vi "Lab Panel V5.22.1.vi"() -> ()   [LabVIEW 2013] (continued)
                                n836 = Number To Decimal String(number=w1475) -> (decimal integer string=w1488:string)  [unwired: 1 in]
                                n837 = Build Array(w1479, w1478, w1490, w1489, w1488) -> (w1487:string[])
                                n838 = TDMS Set Properties(5:w1487, 7:w1481, 11:w1491) -> ()  [unwired: 3 in, 4 out]
                              }
                              frame #3 {
                                n839 = local read "DISP LAB03-2"() -> (w1496:T4)
                                n840 = Concatenate Strings("LAB03-2  ", w1495) -> (w1497:string)
                                n841 = Two Button Dialog(message=w1497, 1:w1493, 2:w1494) -> (T button?=w1499:bool)
                                n842 = case shown="True" w1499 {
                                tunnel: w1496 -> [w1506 w1507]
                                tunnel: [w1506 w1507] -> w1503
                                tunnel: [w1505 w1508] -> w1502
                                tunnel: [w1504 w1508] -> w1501
                                frame False {
                                n843 = Unbundle(w1506) -> ("CYCLE"=w1505:dbl, "MINS"=w1504:dbl)  [unwired: 1 out]
                                }
                                frame True {
                                w1508 = 0.0
                                }
                                }
                                n844 = Bundle(cluster=w1503, "CYCLE"=w1502, "MINS"=w1501, "STATUS"="RUN") -> (w1492:T4)
                                n845 = local write "DISP LAB03-2"(w1492) -> ()
                              }
                              frame #4 {
                                n846 = local read "TEMP START LAB03-2"() -> (w1511:cluster{"TL":dbl, "TN":dbl})
                                n847 = Bundle(cluster=w1511, "TL"=w1509, "TN"=w1509) -> (w1510:cluster{"TL":dbl, "TN":dbl})
                                n848 = local write "TEMP START LAB03-2"(w1510) -> ()
                              }
                            }
                          }
                        }
                      }
                    }
                  }
                }
              }
              event "RUN LAB04-1": Value Change {
                n849 = event-data() -> ("NewVal"=w1516:bool)  [unwired: 1 in, 5 out]
                n850 = local write "run lab04-1"(w1516) -> ()
                n851 = case shown="True" w1516 {
                  tunnel: w1522 -> [_ w1560]
                  tunnel: w1521 -> [_ w1559]
                  tunnel: w1519 -> [w1524 w1558]
                  tunnel: w1520 -> [_ w1557]
                  tunnel: w1518 -> [_ w1556]
                  tunnel: [w1523 w1555] -> w1517
                  tunnel: w1515 -> [_ w1554]
                  tunnel: w1514 -> [_ w1553]
                  tunnel: w1513 -> [_ w1552]
                  tunnel: w1512 -> [_ w1550]
                  frame False {
                    # "stop test"
                    n852 = stacked-sequence {
                      tunnel: w1524 -> [w1533 _]
                      tunnel: [w1525 _] -> w1523
                      frame #0 {
                        n853 = local read "DISP LAB04-1"() -> (w1532:T4)
                        n854 = Unbundle(w1532) -> ("CYCLE"=w1530:dbl, "MINS"=w1531:dbl)  [unwired: 1 out]
                        n855 = case shown="\"CYCLE TEST\"" w1533 {
                          tunnel: w1531 -> [_ _ w1540]
                          tunnel: w1530 -> [w1538 w1539 _]
                          tunnel: [w1538 w1539 w1540] -> w1529
                          frame "CHART TEST", Default {
                          }
                          frame "CYCLE TEST" {
                          }
                          frame "T-RISE TEST" {
                          }
                        }
                        n856 = local read "TDMS LAB04-1"() -> (w1537:refnum<k34>)
                        n857 = Build Array("STOPPED") -> (w1534:string[])
                        n858 = Build Array(w1529) -> (w1528:dbl[])
                        n859 = TDMS Write(0:w1537, 5:"TEST RESULT", 7:w1534, 9:w1528) -> (4:w1526:refnum<k34>, 15:w1527:errorcluster)  [unwired: 2 in, 2 out]
                        n860 = TDMS Close(8:w1527, 11:w1526) -> (0:w1525:errorcluster)  [unwired: 1 out]
                      }
                      frame #1 {
                        n861 = local read "DISP LAB04-1"() -> (w1544:T4)
                        n862 = stacked-sequence {
                          tunnel: "LAB04-1" -> [w1546 w1548]
                          frame #0 {
                            n863 = call "sub vi - defrag tdms v1.vi"("panel id"=w1546) -> ("error out"=w1545:errorcluster)  [unwired: 10 in]
                            n864 = local write "data file error"(w1545) -> ()
                          }
                          frame #1 {
                            n865 = call "Save data file (stop) v3.vi"("panel id"=w1548) -> ("network file save error"=w1547:errorcluster)  [unwired: 9 in, 1 out]
                            n866 = local write "RESULT LAB04-1"(FALSE) -> ()
                            n867 = local write "data file error"(w1547) -> ()
                          }
                        }
                        n868 = Bundle(cluster=w1544, "STATUS"="STOP") -> (w1542:T4)  [unwired: 2 in]
                        n869 = local write "DISP LAB04-1"(w1542) -> ()
                      }
                    }
                  }
                  frame True {
                    n870 = local read "SIG LAB04-1"() -> (w1551:T2)
                    n871 = stacked-sequence {
                      seq-local: [w1562 _] -> [_ w1566]
                      tunnel: w1560 -> [_ w1576]
                      tunnel: w1559 -> [_ w1575]
                      tunnel: w1558 -> [_ w1574]
                      tunnel: w1557 -> [_ w1573]
                      tunnel: w1556 -> [_ w1572]
                      tunnel: [_ w1571] -> w1555
                      tunnel: w1554 -> [_ w1570]
                      tunnel: w1553 -> [_ w1569]
                      tunnel: w1552 -> [_ w1568]
                      tunnel: w1551 -> [w1561 w1567]
                      tunnel: w1550 -> [_ w1565]
                      frame #0 {
                        n872 = Unbundle(w1561) -> ("AMPS"=w1564:dbl)  [unwired: 4 out]
                        n873 = call "Check For Amps on v1.vi"("ID"="LAB04-1", "amps"=w1564) -> ("amps"=w1562:bool)  [unwired: 9 in]
                      }
                      frame #1 {
                        n874 = case shown="True" w1566 {
                          tunnel: w1576 -> [_ w1589]
                          tunnel: w1575 -> [_ w1588]
                          tunnel: w1574 -> [_ w1587]
                          tunnel: w1573 -> [_ w1586]
                          tunnel: w1572 -> [_ w1585]
                          tunnel: [errorcluster {"status"=FALSE, "code"=0, "source"=""} ("error out") w1584] -> w1571
                          tunnel: w1570 -> [_ w1583]
                          tunnel: w1569 -> [_ w1582]
                          tunnel: w1568 -> [_ w1581]
                          tunnel: w1567 -> [_ w1580]
                          tunnel: w1565 -> [_ w1579]
                          frame False {
                            w1577 = FALSE
                            n875 = local write "RUN LAB04-1"(w1577) -> ()
                            n876 = local write "run lab04-1"(w1577) -> ()
                          }
                          frame True {
                            n877 = stacked-sequence {
                              seq-local: [w1590 _ _ _ _] -> [_ w1614 _ _ _]
                              tunnel: w1589 -> [w1595 _ _ _ _]
                              tunnel: w1588 -> [w1591 _ _ _ _]
                              tunnel: w1587 -> [w1605 _ _ _ _]
                              tunnel: w1586 -> [w1598 _ _ _ _]
                              tunnel: w1585 -> [w1593 _ _ _ _]
                              tunnel: [_ w1609 _ _ _] -> w1584
                              tunnel: w1583 -> [_ _ _ w1635 _]
                              tunnel: w1582 -> [_ _ _ w1634 _]
                              tunnel: w1581 -> [_ _ _ w1633 _]
                              tunnel: w1580 -> [_ _ _ _ _]
                              tunnel: w1579 -> [_ _ _ _ w1649]
                              frame #0 {
                                w1592 = "\\"
                                n878 = local read "SET LAB04-1"() -> (w1600:T5)
                                n879 = case shown="\"CYCLE TEST\"" w1605 {
                                tunnel: ["L04-1-CHART TEST-" "L04-1-CYCLE TEST-" "L04-1-T-RISE TEST-"] -> w1601
                                frame "CHART TEST", Default {
                                }
                                frame "CYCLE TEST" {
                                }
                                frame "T-RISE TEST" {
                                }
                                }
                                n880 = Unbundle(w1600) -> ("DESCRIPTION"=w1599:string)  [unwired: 4 out]
                                n881 = Concatenate Strings(w1595, "\\", w1593, w1592, w1591, w1592) -> (w1602:string)
                                n882 = String To Path(string=w1602) -> (path=w1604:path)
                                n883 = Concatenate Strings(w1602, w1601, w1599, "-", w1598, ".tdms") -> (w1590:string)
                                n884 = Create Folder(path (use dialog)=w1604) -> (error out=w1603:errorcluster)  [unwired: 2 in, 2 out]
                                n885 = global write "Global 1.vi" "LAB04-1 FILE"(w1590) -> ()
                                n886 = call <vilib>:"Clear Errors.vi"("error in (no error)"=w1603) -> ()  [unwired: 6 in, 1 out]
                              }
                              frame #1 {
                                (unwired) FALSE
                                n887 = String To Path(string=w1614) -> (path=w1610:path)
                                n888 = TDMS Open(6:FALSE, 10:T21."create or replace" ("operation (0:open)"), 11:w1610) -> (0:w1609:errorcluster, 3:→"TDMS LAB04-1":refnum<k34>)  [unwired: 4 in]
                              }
                              frame #2 {
                                n889 = local read "SET LAB04-1"() -> (w1620:T5)
                                n890 = local read "TDMS LAB04-1"() -> (w1631:refnum<k34>)
                                n891 = Build Array("Testers Name", "Description", "Set Test Cycles", "T-Rise minutes", "T-Rise Deg C") -> (w1621:string[])
                                n892 = Unbundle(w1620) -> ("NAME"=w1619:string, "DESCRIPTION"=w1618:string, "CYCLES"=w1617:dbl, "T-RISE mins"=w1616:dbl, "T-RISE deg C"=w1615:dbl)
                                n893 = Number To Decimal String(number=w1617) -> (decimal integer string=w1630:string)  [unwired: 1 in]
                                n894 = Number To Decimal String(number=w1616) -> (decimal integer string=w1629:string)  [unwired: 1 in]
                                n895 = Number To Decimal String(number=w1615) -> (decimal integer string=w1628:string)  [unwired: 1 in]
                                n896 = Build Array(w1619, w1618, w1630, w1629, w1628) -> (w1627:string[])
                                n897 = TDMS Set Properties(5:w1627, 7:w1621, 11:w1631) -> ()  [unwired: 3 in, 4 out]
                              }
                              frame #3 {
                                n898 = local read "DISP LAB04-1"() -> (w1636:T4)
                                n899 = Concatenate Strings("LAB04-1  ", w1635) -> (w1637:string)
                                n900 = Two Button Dialog(message=w1637, 1:w1633, 2:w1634) -> (T button?=w1639:bool)
                                n901 = case shown="True" w1639 {
                                tunnel: w1636 -> [w1646 w1647]
                                tunnel: [w1646 w1647] -> w1643
                                tunnel: [w1645 w1648] -> w1642
                                tunnel: [w1644 w1648] -> w1641
                                frame False {
                                n902 = Unbundle(w1646) -> ("CYCLE"=w1645:dbl, "MINS"=w1644:dbl)  [unwired: 1 out]
                                }
                                frame True {
                                w1648 = 0.0
                                }
                                }
                                n903 = Bundle(cluster=w1643, "CYCLE"=w1642, "MINS"=w1641, "STATUS"="RUN") -> (w1632:T4)
                                n904 = local write "DISP LAB04-1"(w1632) -> ()
                              }
                              frame #4 {
                                n905 = local read "TEMP START LAB04-1"() -> (w1651:cluster{"TL":dbl, "TN":dbl})
                                n906 = Bundle(cluster=w1651, "TL"=w1649, "TN"=w1649) -> (w1650:cluster{"TL":dbl, "TN":dbl})
                                n907 = local write "TEMP START LAB04-1"(w1650) -> ()
                              }
                            }
                          }
                        }
                      }
                    }
                  }
                }
              }
              event "RUN LAB04-2": Value Change {
                n908 = event-data() -> ("NewVal"=w1656:bool)  [unwired: 1 in, 5 out]
                n909 = local write "run lab04-2"(w1656) -> ()
                n910 = case shown="True" w1656 {
                  tunnel: w1662 -> [_ w1700]
                  tunnel: w1661 -> [_ w1699]
                  tunnel: w1659 -> [w1664 w1698]
                  tunnel: w1660 -> [_ w1697]
                  tunnel: w1658 -> [_ w1696]
                  tunnel: [w1663 w1695] -> w1657
                  tunnel: w1655 -> [_ w1694]
                  tunnel: w1654 -> [_ w1693]
                  tunnel: w1653 -> [_ w1692]
                  tunnel: w1652 -> [_ w1690]
                  frame False {
                    # "stop test"
                    n911 = stacked-sequence {
                      tunnel: w1664 -> [w1673 _]
                      tunnel: [w1665 _] -> w1663
                      frame #0 {
                        n912 = local read "DISP LAB04-2"() -> (w1672:T4)
                        n913 = Unbundle(w1672) -> ("CYCLE"=w1670:dbl, "MINS"=w1671:dbl)  [unwired: 1 out]
                        n914 = case shown="\"CYCLE TEST\"" w1673 {
                          tunnel: w1671 -> [_ _ w1680]
                          tunnel: w1670 -> [w1678 w1679 _]
                          tunnel: [w1678 w1679 w1680] -> w1669
                          frame "CHART TEST", Default {
                          }
                          frame "CYCLE TEST" {
                          }
                          frame "T-RISE TEST" {
                          }
                        }
                        n915 = local read "TDMS LAB04-2"() -> (w1677:refnum<k34>)
                        n916 = Build Array("STOPPED") -> (w1674:string[])
                        n917 = Build Array(w1669) -> (w1668:dbl[])
                        n918 = TDMS Write(0:w1677, 5:"TEST RESULT", 7:w1674, 9:w1668) -> (4:w1666:refnum<k34>, 15:w1667:errorcluster)  [unwired: 2 in, 2 out]
                        n919 = TDMS Close(8:w1667, 11:w1666) -> (0:w1665:errorcluster)  [unwired: 1 out]
                      }
                      frame #1 {
                        n920 = local read "DISP LAB04-2"() -> (w1684:T4)
                        n921 = stacked-sequence {
                          tunnel: "LAB04-2" -> [w1686 w1688]
                          frame #0 {
                            n922 = call "sub vi - defrag tdms v1.vi"("panel id"=w1686) -> ("error out"=w1685:errorcluster)  [unwired: 10 in]
                            n923 = local write "data file error"(w1685) -> ()
                          }
                          frame #1 {
                            n924 = call "Save data file (stop) v3.vi"("panel id"=w1688) -> ("network file save error"=w1687:errorcluster)  [unwired: 9 in, 1 out]
                            n925 = local write "RESULT LAB04-2"(FALSE) -> ()
                            n926 = local write "data file error"(w1687) -> ()
                          }
                        }
                        n927 = Bundle(cluster=w1684, "STATUS"="STOP") -> (w1682:T4)  [unwired: 2 in]
                        n928 = local write "DISP LAB04-2"(w1682) -> ()
                      }
                    }
                  }
                  frame True {
                    n929 = local read "SIG LAB04-2"() -> (w1691:T2)
                    n930 = stacked-sequence {
                      seq-local: [w1702 _] -> [_ w1706]
                      tunnel: w1700 -> [_ w1716]
                      tunnel: w1699 -> [_ w1715]
                      tunnel: w1698 -> [_ w1714]
                      tunnel: w1697 -> [_ w1713]
                      tunnel: w1696 -> [_ w1712]
                      tunnel: [_ w1711] -> w1695
                      tunnel: w1694 -> [_ w1710]
                      tunnel: w1693 -> [_ w1709]
                      tunnel: w1692 -> [_ w1708]
                      tunnel: w1691 -> [w1701 w1707]
                      tunnel: w1690 -> [_ w1705]
                      frame #0 {
                        n931 = Unbundle(w1701) -> ("AMPS"=w1704:dbl)  [unwired: 4 out]
                        n932 = call "Check For Amps on v1.vi"("ID"="LAB04-2", "amps"=w1704) -> ("amps"=w1702:bool)  [unwired: 9 in]
                      }
                      frame #1 {
                        n933 = case shown="True" w1706 {
                          tunnel: w1716 -> [_ w1729]
                          tunnel: w1715 -> [_ w1728]
                          tunnel: w1714 -> [_ w1727]
                          tunnel: w1713 -> [_ w1726]
                          tunnel: w1712 -> [_ w1725]
                          tunnel: [errorcluster {"status"=FALSE, "code"=0, "source"=""} ("error out") w1724] -> w1711
                          tunnel: w1710 -> [_ w1723]
                          tunnel: w1709 -> [_ w1722]
                          tunnel: w1708 -> [_ w1721]
                          tunnel: w1707 -> [_ w1720]
                          tunnel: w1705 -> [_ w1719]
                          frame False {
                            w1717 = FALSE
                            n934 = local write "RUN LAB04-2"(w1717) -> ()
                            n935 = local write "run lab04-2"(w1717) -> ()
                          }
                          frame True {
                            n936 = stacked-sequence {
                              seq-local: [w1730 _ _ _ _] -> [_ w1754 _ _ _]
                              tunnel: w1729 -> [w1735 _ _ _ _]
                              tunnel: w1728 -> [w1731 _ _ _ _]
                              tunnel: w1727 -> [w1745 _ _ _ _]
                              tunnel: w1726 -> [w1738 _ _ _ _]
                              tunnel: w1725 -> [w1733 _ _ _ _]
                              tunnel: [_ w1749 _ _ _] -> w1724
                              tunnel: w1723 -> [_ _ _ w1775 _]
                              tunnel: w1722 -> [_ _ _ w1774 _]
                              tunnel: w1721 -> [_ _ _ w1773 _]
                              tunnel: w1720 -> [_ _ _ _ _]
                              tunnel: w1719 -> [_ _ _ _ w1789]
                              frame #0 {
                                w1732 = "\\"
                                n937 = local read "SET LAB04-2"() -> (w1740:T5)
                                n938 = case shown="\"CHART TEST\", Default" w1745 {
                                tunnel: ["L04-2-CHART TEST-" "L04-2-CYCLE TEST-" "L04-2-T-RISE TEST-"] -> w1741
                                frame "CHART TEST", Default {
                                }
                                frame "CYCLE TEST" {
                                }
                                frame "T-RISE TEST" {
                                }
                                }
                                n939 = Unbundle(w1740) -> ("DESCRIPTION"=w1739:string)  [unwired: 4 out]
                                n940 = Concatenate Strings(w1735, "\\", w1733, w1732, w1731, w1732) -> (w1742:string)
                                n941 = String To Path(string=w1742) -> (path=w1744:path)
                                n942 = Concatenate Strings(w1742, w1741, w1739, "-", w1738, ".tdms") -> (w1730:string)
                                n943 = Create Folder(path (use dialog)=w1744) -> (error out=w1743:errorcluster)  [unwired: 2 in, 2 out]
                                n944 = global write "Global 1.vi" "LAB04-2 FILE"(w1730) -> ()
                                n945 = call <vilib>:"Clear Errors.vi"("error in (no error)"=w1743) -> ()  [unwired: 6 in, 1 out]
                              }
                              frame #1 {
                                (unwired) FALSE
                                n946 = String To Path(string=w1754) -> (path=w1750:path)
                                n947 = TDMS Open(6:FALSE, 10:T21."create or replace" ("operation (0:open)"), 11:w1750) -> (0:w1749:errorcluster, 3:→"TDMS LAB04-2":refnum<k34>)  [unwired: 4 in]
                              }
                              frame #2 {
                                n948 = local read "SET LAB04-2"() -> (w1760:T5)
                                n949 = local read "TDMS LAB04-2"() -> (w1771:refnum<k34>)
                                n950 = Build Array("Testers Name", "Description", "Set Test Cycles", "T-Rise minutes", "T-Rise Deg C") -> (w1761:string[])
                                n951 = Unbundle(w1760) -> ("NAME"=w1759:string, "DESCRIPTION"=w1758:string, "CYCLES"=w1757:dbl, "T-RISE mins"=w1756:dbl, "T-RISE deg C"=w1755:dbl)
                                n952 = Number To Decimal String(number=w1757) -> (decimal integer string=w1770:string)  [unwired: 1 in]
                                n953 = Number To Decimal String(number=w1756) -> (decimal integer string=w1769:string)  [unwired: 1 in]
                                n954 = Number To Decimal String(number=w1755) -> (decimal integer string=w1768:string)  [unwired: 1 in]
                                n955 = Build Array(w1759, w1758, w1770, w1769, w1768) -> (w1767:string[])
                                n956 = TDMS Set Properties(5:w1767, 7:w1761, 11:w1771) -> ()  [unwired: 3 in, 4 out]
                              }
                              frame #3 {
                                n957 = local read "DISP LAB04-2"() -> (w1776:T4)
                                n958 = Concatenate Strings("LAB04-2 ", w1775) -> (w1777:string)
                                n959 = Two Button Dialog(message=w1777, 1:w1773, 2:w1774) -> (T button?=w1779:bool)
                                n960 = case shown="True" w1779 {
                                tunnel: w1776 -> [w1786 w1787]
                                tunnel: [w1786 w1787] -> w1783
                                tunnel: [w1785 w1788] -> w1782
                                tunnel: [w1784 w1788] -> w1781
                                frame False {
                                n961 = Unbundle(w1786) -> ("CYCLE"=w1785:dbl, "MINS"=w1784:dbl)  [unwired: 1 out]
                                }
                                frame True {
                                w1788 = 0.0
                                }
                                }
                                n962 = Bundle(cluster=w1783, "CYCLE"=w1782, "MINS"=w1781, "STATUS"="RUN") -> (w1772:T4)
                                n963 = local write "DISP LAB04-2"(w1772) -> ()
                              }
                              frame #4 {
                                n964 = local read "TEMP START LAB04-2"() -> (w1791:cluster{"TL":dbl, "TN":dbl})
                                n965 = Bundle(cluster=w1791, "TL"=w1789, "TN"=w1789) -> (w1790:cluster{"TL":dbl, "TN":dbl})
                                n966 = local write "TEMP START LAB04-2"(w1790) -> ()
                              }
                            }
                          }
                        }
                      }
                    }
                  }
                }
              }
              event "RUN LAB05-1": Value Change {
                n967 = event-data() -> ("NewVal"=w1796:bool)  [unwired: 1 in, 5 out]
                n968 = local write "run lab05-1"(w1796) -> ()
                n969 = case shown="True" w1796 {
                  tunnel: w1802 -> [_ w1840]
                  tunnel: w1801 -> [_ w1839]
                  tunnel: w1799 -> [w1804 w1838]
                  tunnel: w1800 -> [_ w1837]
                  tunnel: w1798 -> [_ w1836]
                  tunnel: [w1803 w1835] -> w1797
                  tunnel: w1795 -> [_ w1834]
                  tunnel: w1794 -> [_ w1833]
                  tunnel: w1793 -> [_ w1832]
                  tunnel: w1792 -> [_ w1830]
                  frame False {
                    # "stop test"
                    n970 = stacked-sequence {
                      tunnel: w1804 -> [w1813 _]
                      tunnel: [w1805 _] -> w1803
                      frame #0 {
                        n971 = local read "DISP LAB05-1"() -> (w1812:T4)
                        n972 = Unbundle(w1812) -> ("CYCLE"=w1810:dbl, "MINS"=w1811:dbl)  [unwired: 1 out]
                        n973 = case shown="\"CYCLE TEST\"" w1813 {
                          tunnel: w1811 -> [_ _ w1820]
                          tunnel: w1810 -> [w1818 w1819 _]
                          tunnel: [w1818 w1819 w1820] -> w1809
                          frame "CHART TEST", Default {
                          }
                          frame "CYCLE TEST" {
                          }
                          frame "T-RISE TEST" {
                          }
                        }
                        n974 = local read "TDMS LAB05-1"() -> (w1817:refnum<k34>)
                        n975 = Build Array("STOPPED") -> (w1814:string[])
                        n976 = Build Array(w1809) -> (w1808:dbl[])
                        n977 = TDMS Write(0:w1817, 5:"TEST RESULT", 7:w1814, 9:w1808) -> (4:w1806:refnum<k34>, 15:w1807:errorcluster)  [unwired: 2 in, 2 out]
                        n978 = TDMS Close(8:w1807, 11:w1806) -> (0:w1805:errorcluster)  [unwired: 1 out]
                      }
                      frame #1 {
                        n979 = local read "DISP LAB05-1"() -> (w1824:T4)
                        n980 = stacked-sequence {
                          tunnel: "LAB05-1" -> [w1826 w1828]
                          frame #0 {
                            n981 = call "sub vi - defrag tdms v1.vi"("panel id"=w1826) -> ("error out"=w1825:errorcluster)  [unwired: 10 in]
                            n982 = local write "data file error"(w1825) -> ()
                          }
                          frame #1 {
                            n983 = call "Save data file (stop) v3.vi"("panel id"=w1828) -> ("network file save error"=w1827:errorcluster)  [unwired: 9 in, 1 out]
                            n984 = local write "RESULT LAB05-1"(FALSE) -> ()
                            n985 = local write "data file error"(w1827) -> ()
                          }
                        }
                        n986 = Bundle(cluster=w1824, "STATUS"="STOP") -> (w1822:T4)  [unwired: 2 in]
                        n987 = local write "DISP LAB05-1"(w1822) -> ()
                      }
                    }
                  }
                  frame True {
                    n988 = local read "SIG LAB05-1"() -> (w1831:T2)
                    n989 = stacked-sequence {
                      seq-local: [w1842 _] -> [_ w1846]
                      tunnel: w1840 -> [_ w1856]
                      tunnel: w1839 -> [_ w1855]
                      tunnel: w1838 -> [_ w1854]
                      tunnel: w1837 -> [_ w1853]
                      tunnel: w1836 -> [_ w1852]
                      tunnel: [_ w1851] -> w1835
                      tunnel: w1834 -> [_ w1850]
                      tunnel: w1833 -> [_ w1849]
                      tunnel: w1832 -> [_ w1848]
                      tunnel: w1831 -> [w1841 w1847]
                      tunnel: w1830 -> [_ w1845]
                      frame #0 {
                        n990 = Unbundle(w1841) -> ("AMPS"=w1844:dbl)  [unwired: 4 out]
                        n991 = call "Check For Amps on v1.vi"("ID"="LAB05-1", "amps"=w1844) -> ("amps"=w1842:bool)  [unwired: 9 in]
                      }
                      frame #1 {
                        n992 = case shown="True" w1846 {
                          tunnel: w1856 -> [_ w1869]
                          tunnel: w1855 -> [_ w1868]
                          tunnel: w1854 -> [_ w1867]
                          tunnel: w1853 -> [_ w1866]
                          tunnel: w1852 -> [_ w1865]
                          tunnel: [errorcluster {"status"=FALSE, "code"=0, "source"=""} ("error out") w1864] -> w1851
                          tunnel: w1850 -> [_ w1863]
                          tunnel: w1849 -> [_ w1862]
                          tunnel: w1848 -> [_ w1861]
                          tunnel: w1847 -> [_ w1860]
                          tunnel: w1845 -> [_ w1859]
                          frame False {
                            w1857 = FALSE
                            n993 = local write "RUN LAB05-1"(w1857) -> ()
                            n994 = local write "run lab05-1"(w1857) -> ()
                          }
                          frame True {
                            n995 = stacked-sequence {
                              seq-local: [w1870 _ _ _ _] -> [_ w1894 _ _ _]
                              tunnel: w1869 -> [w1875 _ _ _ _]
                              tunnel: w1868 -> [w1871 _ _ _ _]
                              tunnel: w1867 -> [w1885 _ _ _ _]
                              tunnel: w1866 -> [w1878 _ _ _ _]
                              tunnel: w1865 -> [w1873 _ _ _ _]
                              tunnel: [_ w1889 _ _ _] -> w1864
                              tunnel: w1863 -> [_ _ _ w1914 _]
                              tunnel: w1862 -> [_ _ _ w1913 _]
                              tunnel: w1861 -> [_ _ _ w1912 _]
                              tunnel: w1860 -> [_ _ _ _ _]
                              tunnel: w1859 -> [_ _ _ _ w1929]
                              frame #0 {
                                w1872 = "\\"
                                n996 = local read "SET LAB05-1"() -> (w1880:T5)
                                n997 = case shown="\"CYCLE TEST\"" w1885 {
                                tunnel: ["L05-1-CHART TEST-" "L05-1-CYCLE TEST-" "L05-1-T-RISE TEST-"] -> w1881
                                frame "CHART TEST", Default {
                                }
                                frame "CYCLE TEST" {
                                }
                                frame "T-RISE TEST" {
                                }
                                }
                                n998 = Unbundle(w1880) -> ("DESCRIPTION"=w1879:string)  [unwired: 4 out]
                                n999 = Concatenate Strings(w1875, "\\", w1873, w1872, w1871, w1872) -> (w1882:string)
                                n1000 = String To Path(string=w1882) -> (path=w1884:path)
                                n1001 = Concatenate Strings(w1882, w1881, w1879, "-", w1878, ".tdms") -> (w1870:string)
                                n1002 = Create Folder(path (use dialog)=w1884) -> (error out=w1883:errorcluster)  [unwired: 2 in, 2 out]
                                n1003 = global write "Global 1.vi" "LAB05-1 FILE"(w1870) -> ()
                                n1004 = call <vilib>:"Clear Errors.vi"("error in (no error)"=w1883) -> ()  [unwired: 6 in, 1 out]
                              }
                              frame #1 {
                                (unwired) FALSE
                                n1005 = String To Path(string=w1894) -> (path=w1890:path)
                                n1006 = TDMS Open(6:FALSE, 10:T21."create or replace" ("operation (0:open)"), 11:w1890) -> (0:w1889:errorcluster, 3:→"TDMS LAB05-1":refnum<k34>)  [unwired: 4 in]
                              }
                              frame #2 {
                                n1007 = local read "SET LAB05-1"() -> (w1900:T5)
                                n1008 = local read "TDMS LAB05-1"() -> (w1911:refnum<k34>)
                                n1009 = Build Array("Testers Name", "Description", "Set Test Cycles", "T-Rise minutes", "T-Rise Deg C") -> (w1901:string[])
                                n1010 = Unbundle(w1900) -> ("NAME"=w1899:string, "DESCRIPTION"=w1898:string, "CYCLES"=w1897:dbl, "T-RISE mins"=w1896:dbl, "T-RISE deg C"=w1895:dbl)
                                n1011 = Number To Decimal String(number=w1897) -> (decimal integer string=w1910:string)  [unwired: 1 in]
                                n1012 = Number To Decimal String(number=w1896) -> (decimal integer string=w1909:string)  [unwired: 1 in]
                                n1013 = Number To Decimal String(number=w1895) -> (decimal integer string=w1908:string)  [unwired: 1 in]
                                n1014 = Build Array(w1899, w1898, w1910, w1909, w1908) -> (w1907:string[])
                                n1015 = TDMS Set Properties(5:w1907, 7:w1901, 11:w1911) -> ()  [unwired: 3 in, 4 out]
                              }
                              frame #3 {
                                n1016 = local read "DISP LAB05-1"() -> (w1916:T4)
                                n1017 = Concatenate Strings("LAB05-1  ", w1914) -> (w1917:string)
                                n1018 = Two Button Dialog(message=w1917, 1:w1912, 2:w1913) -> (T button?=w1919:bool)
                                n1019 = case shown="True" w1919 {
                                tunnel: w1916 -> [w1926 w1927]
                                tunnel: [w1926 w1927] -> w1923
                                tunnel: [w1925 w1928] -> w1922
                                tunnel: [w1924 w1928] -> w1921
                                frame False {
                                n1020 = Unbundle(w1926) -> ("CYCLE"=w1925:dbl, "MINS"=w1924:dbl)  [unwired: 1 out]
                                }
                                frame True {
                                w1928 = 0.0
                                }
                                }
                                n1021 = Bundle(cluster=w1923, "CYCLE"=w1922, "MINS"=w1921, "STATUS"="RUN") -> (w1915:T4)
                                n1022 = local write "DISP LAB05-1"(w1915) -> ()
                              }
                              frame #4 {
                                n1023 = local read "TEMP START LAB05-1"() -> (w1931:cluster{"TL":dbl, "TN":dbl})
                                n1024 = Bundle(cluster=w1931, "TL"=w1929, "TN"=w1929) -> (w1930:cluster{"TL":dbl, "TN":dbl})
                                n1025 = local write "TEMP START LAB05-1"(w1930) -> ()
                              }
                            }
                          }
                        }
                      }
                    }
                  }
                }
              }
              event "RUN LAB05-2": Value Change {
                n1026 = event-data() -> ("NewVal"=w1937:bool)  [unwired: 1 in, 5 out]
                n1027 = local read "SIG LAB05-2"() -> (w1933:T2)
                n1028 = case shown="True" w1937 {
                  tunnel: w1943 -> [_ w1981]
                  tunnel: w1942 -> [_ w1980]
                  tunnel: w1940 -> [w1945 w1979]
                  tunnel: w1941 -> [_ w1978]
                  tunnel: w1939 -> [_ w1977]
                  tunnel: [w1944 w1976] -> w1938
                  tunnel: w1936 -> [_ w1975]
                  tunnel: w1935 -> [_ w1974]
                  tunnel: w1934 -> [_ w1973]
                  tunnel: w1933 -> [_ w1972]
                  tunnel: w1932 -> [_ w1971]
                  frame False {
                    # "stop test"
                    n1029 = stacked-sequence {
                      tunnel: w1945 -> [w1954 _]
                      tunnel: [w1946 _] -> w1944
                      frame #0 {
                        n1030 = local read "DISP LAB05-2"() -> (w1953:T4)
                        n1031 = Unbundle(w1953) -> ("CYCLE"=w1951:dbl, "MINS"=w1952:dbl)  [unwired: 1 out]
                        n1032 = case shown="\"CYCLE TEST\"" w1954 {
                          tunnel: w1952 -> [_ _ w1961]
                          tunnel: w1951 -> [w1959 w1960 _]
                          tunnel: [w1959 w1960 w1961] -> w1950
                          frame "CHART TEST", Default {
                          }
                          frame "CYCLE TEST" {
                          }
                          frame "T-RISE TEST" {
                          }
                        }
                        n1033 = local read "TDMS LAB05-2"() -> (w1958:refnum<k34>)
                        n1034 = Build Array("STOPPED") -> (w1955:string[])
                        n1035 = Build Array(w1950) -> (w1949:dbl[])
                        n1036 = TDMS Write(0:w1958, 5:"TEST RESULT", 7:w1955, 9:w1949) -> (4:w1947:refnum<k34>, 15:w1948:errorcluster)  [unwired: 2 in, 2 out]
                        n1037 = TDMS Close(8:w1948, 11:w1947) -> (0:w1946:errorcluster)  [unwired: 1 out]
                      }
                      frame #1 {
                        n1038 = local read "DISP LAB05-2"() -> (w1965:T4)
                        n1039 = stacked-sequence {
                          tunnel: "LAB05-2" -> [w1967 w1969]
                          frame #0 {
                            n1040 = call "sub vi - defrag tdms v1.vi"("panel id"=w1967) -> ("error out"=w1966:errorcluster)  [unwired: 10 in]
                            n1041 = local write "data file error"(w1966) -> ()
                          }
                          frame #1 {
                            n1042 = local write "RESULT LAB05-2"(FALSE) -> ()
                            n1043 = call "Save data file (stop) v3.vi"("panel id"=w1969) -> ("network file save error"=w1968:errorcluster)  [unwired: 9 in, 1 out]
                            n1044 = local write "data file error"(w1968) -> ()
                          }
                        }
                        n1045 = Bundle(cluster=w1965, "STATUS"="STOP") -> (w1963:T4)  [unwired: 2 in]
                        n1046 = local write "DISP LAB05-2"(w1963) -> ()
                      }
                    }
                  }
                  frame True {
                    n1047 = stacked-sequence {
                      seq-local: [w1983 _] -> [_ w1987]
                      tunnel: w1981 -> [_ w1997]
                      tunnel: w1980 -> [_ w1996]
                      tunnel: w1979 -> [_ w1995]
                      tunnel: w1978 -> [_ w1994]
                      tunnel: w1977 -> [_ w1993]
                      tunnel: [_ w1992] -> w1976
                      tunnel: w1975 -> [_ w1991]
                      tunnel: w1974 -> [_ w1990]
                      tunnel: w1973 -> [_ w1989]
                      tunnel: w1972 -> [w1982 w1988]
                      tunnel: w1971 -> [_ w1986]
                      frame #0 {
                        n1048 = Unbundle(w1982) -> ("AMPS"=w1985:dbl)  [unwired: 4 out]
                        n1049 = call "Check For Amps on v1.vi"("ID"="LAB05-2", "amps"=w1985) -> ("amps"=w1983:bool)  [unwired: 9 in]
                      }
                      frame #1 {
                        n1050 = case shown="True" w1987 {
                          tunnel: w1997 -> [_ w2010]
                          tunnel: w1996 -> [_ w2009]
                          tunnel: w1995 -> [_ w2008]
                          tunnel: w1994 -> [_ w2007]
                          tunnel: w1993 -> [_ w2006]
                          tunnel: [errorcluster {"status"=FALSE, "code"=0, "source"=""} ("error out") w2005] -> w1992
                          tunnel: w1991 -> [_ w2004]
                          tunnel: w1990 -> [_ w2003]
                          tunnel: w1989 -> [_ w2002]
                          tunnel: w1988 -> [_ w2001]
                          tunnel: w1986 -> [_ w2000]
                          frame False {
                            w1998 = FALSE
                            n1051 = local write "RUN LAB05-2"(w1998) -> ()
                            n1052 = local write "run lab05-2"(w1998) -> ()
                          }
                          frame True {
                            n1053 = stacked-sequence {
                              seq-local: [w2011 _ _ _ _] -> [_ w2035 _ _ _]
                              tunnel: w2010 -> [w2016 _ _ _ _]
                              tunnel: w2009 -> [w2012 _ _ _ _]
                              tunnel: w2008 -> [w2026 _ _ _ _]
                              tunnel: w2007 -> [w2019 _ _ _ _]
                              tunnel: w2006 -> [w2014 _ _ _ _]
                              tunnel: [_ w2030 _ _ _] -> w2005
                              tunnel: w2004 -> [_ _ _ w2055 _]
                              tunnel: w2003 -> [_ _ _ w2054 _]
                              tunnel: w2002 -> [_ _ _ w2053 _]
                              tunnel: w2001 -> [_ _ _ _ _]
                              tunnel: w2000 -> [_ _ _ _ w2070]
                              frame #0 {
                                w2013 = "\\"
                                n1054 = local read "SET LAB05-2"() -> (w2021:T5)
                                n1055 = case shown="\"CYCLE TEST\"" w2026 {
                                tunnel: ["L05-2-CHART TEST-" "L05-2-CYCLE TEST-" "L05-2-T-RISE TEST-"] -> w2022
                                frame "CHART TEST", Default {
                                }
                                frame "CYCLE TEST" {
                                }
                                frame "T-RISE TEST" {
                                }
                                }
                                n1056 = Unbundle(w2021) -> ("DESCRIPTION"=w2020:string)  [unwired: 4 out]
                                n1057 = Concatenate Strings(w2016, "\\", w2014, w2013, w2012, w2013) -> (w2023:string)
                                n1058 = String To Path(string=w2023) -> (path=w2025:path)
                                n1059 = Concatenate Strings(w2023, w2022, w2020, "-", w2019, ".tdms") -> (w2011:string)
                                n1060 = Create Folder(path (use dialog)=w2025) -> (error out=w2024:errorcluster)  [unwired: 2 in, 2 out]
                                n1061 = global write "Global 1.vi" "LAB05-2 FILE"(w2011) -> ()
                                n1062 = call <vilib>:"Clear Errors.vi"("error in (no error)"=w2024) -> ()  [unwired: 6 in, 1 out]
                              }
                              frame #1 {
                                (unwired) FALSE
                                n1063 = String To Path(string=w2035) -> (path=w2031:path)
                                n1064 = TDMS Open(6:FALSE, 10:T21."create or replace" ("operation (0:open)"), 11:w2031) -> (0:w2030:errorcluster, 3:→"TDMS LAB05-2":refnum<k34>)  [unwired: 4 in]
                              }
                              frame #2 {
                                n1065 = local read "SET LAB05-2"() -> (w2041:T5)
                                n1066 = local read "TDMS LAB05-2"() -> (w2052:refnum<k34>)
                                n1067 = Build Array("Testers Name", "Description", "Set Test Cycles", "T-Rise minutes", "T-Rise Deg C") -> (w2042:string[])
                                n1068 = Unbundle(w2041) -> ("NAME"=w2040:string, "DESCRIPTION"=w2039:string, "CYCLES"=w2038:dbl, "T-RISE mins"=w2037:dbl, "T-RISE deg C"=w2036:dbl)
                                n1069 = Number To Decimal String(number=w2038) -> (decimal integer string=w2051:string)  [unwired: 1 in]
                                n1070 = Number To Decimal String(number=w2037) -> (decimal integer string=w2050:string)  [unwired: 1 in]
                                n1071 = Number To Decimal String(number=w2036) -> (decimal integer string=w2049:string)  [unwired: 1 in]
                                n1072 = Build Array(w2040, w2039, w2051, w2050, w2049) -> (w2048:string[])
                                n1073 = TDMS Set Properties(5:w2048, 7:w2042, 11:w2052) -> ()  [unwired: 3 in, 4 out]
                              }
                              frame #3 {
                                n1074 = local read "DISP LAB05-2"() -> (w2057:T4)
                                n1075 = Concatenate Strings("LAB05-2  ", w2055) -> (w2058:string)
                                n1076 = Two Button Dialog(message=w2058, 1:w2053, 2:w2054) -> (T button?=w2060:bool)
                                n1077 = case shown="True" w2060 {
                                tunnel: w2057 -> [w2067 w2068]
                                tunnel: [w2067 w2068] -> w2064
                                tunnel: [w2066 w2069] -> w2063
                                tunnel: [w2065 w2069] -> w2062
                                frame False {
                                n1078 = Unbundle(w2067) -> ("CYCLE"=w2066:dbl, "MINS"=w2065:dbl)  [unwired: 1 out]
                                }
                                frame True {
                                w2069 = 0.0
                                }
                                }
                                n1079 = Bundle(cluster=w2064, "CYCLE"=w2063, "MINS"=w2062, "STATUS"="RUN") -> (w2056:T4)
                                n1080 = local write "DISP LAB05-2"(w2056) -> ()
                              }
                              frame #4 {
                                n1081 = local read "TEMP START LAB05-2"() -> (w2072:cluster{"TL":dbl, "TN":dbl})
                                n1082 = Bundle(cluster=w2072, "TL"=w2070, "TN"=w2070) -> (w2071:cluster{"TL":dbl, "TN":dbl})
                                n1083 = local write "TEMP START LAB05-2"(w2071) -> ()
                              }
                            }
                          }
                        }
                      }
                    }
                  }
                }
                n1084 = local write "run lab05-2"(w1937) -> ()
              }
            }
            n1085 = local write "data file error"(w641) -> ()
          }
          frame #4 {
            # "check if test cycles reached for cycle tests, if so then test pass"
            n1086 = stacked-sequence {
              tunnel: w2092 -> [_ _ _ _ _ _ _ _ _ _]
              tunnel: w2091 -> [_ _ _ _ _ _ _ _ _ _]
              tunnel: w2090 -> [_ _ _ _ _ _ _ _ _ _]
              tunnel: w2089 -> [_ _ _ _ _ _ _ _ _ _]
              tunnel: w2088 -> [_ _ _ _ _ _ _ _ _ _]
              tunnel: w2087 -> [_ _ _ _ _ _ _ _ _ _]
              tunnel: w2086 -> [_ _ _ _ _ _ _ _ _ _]
              tunnel: w2085 -> [_ _ _ _ _ _ _ _ _ _]
              tunnel: w2084 -> [_ _ _ _ _ _ _ _ _ _]
              tunnel: w2083 -> [_ _ _ _ _ _ _ _ _ _]
              tunnel: w2082 -> [w2098 _ _ _ _ _ _ _ _ _]
              tunnel: w2081 -> [_ w2133 _ _ _ _ _ _ _ _]
              tunnel: w2080 -> [_ _ w2173 _ _ _ _ _ _ _]
              tunnel: w2079 -> [_ _ _ w2213 _ _ _ _ _ _]
              tunnel: w2078 -> [_ _ _ _ w2253 _ _ _ _ _]
              tunnel: w2077 -> [_ _ _ _ _ w2293 _ _ _ _]
              tunnel: w2076 -> [_ _ _ _ _ _ w2333 _ _ _]
              tunnel: w2075 -> [_ _ _ _ _ _ _ w2373 _ _]
              tunnel: w2074 -> [_ _ _ _ _ _ _ _ w2413 _]
              tunnel: w2073 -> [_ _ _ _ _ _ _ _ _ w2453]
              frame #0 {
                # "LAB01-1"
                n1087 = Less?(x=w2098, y=2) -> (x < y?=w2096:bool)
                n1088 = local read "DISP LAB01-1"() -> (w2099:T4)
                n1089 = Unbundle(w2099) -> ("STATUS"=w2093:string)  [unwired: 2 out]
                n1090 = Equal?(x=w2093, y="RUN") -> (x = y?=w2095:bool)
                n1091 = And(x=w2095, y=w2096) -> (x .and. y?=w2094:bool)
                n1092 = case shown="True" w2094 {
                  tunnel: w2099 -> [_ w2104]
                  tunnel: w2098 -> [_ w2108]
                  frame False {
                  }
                  frame True {
                    n1093 = local read "SET LAB01-1"() -> (w2110:T5)
                    n1094 = local read "TDMS LAB01-1"() -> (w2103:refnum<k34>)
                    n1095 = Unbundle(w2110) -> ("CYCLES"=w2101:dbl, "T-RISE mins"=w2107:dbl)  [unwired: 3 out]
                    n1096 = case shown="\"CYCLE TEST\"" w2108 {
                      tunnel: w2107 -> [_ _ w2117]
                      tunnel: [w2112 w2114 w2117] -> w2106
                      tunnel: w2101 -> [w2112 w2114 _]
                      tunnel: ["CHART PASS" "CYCLE PASS" "T-RISE PASS"] -> w2105
                      frame "CHART TEST", Default {
                      }
                      frame "CYCLE TEST" {
                      }
                      frame "T-RISE TEST" {
                      }
                    }
                    n1097 = Unbundle(w2104) -> ("CYCLE"=w2109:dbl)  [unwired: 2 out]
                    n1098 = Increment(x=w2101) -> (x+1=w2102:dbl)
                    n1099 = Greater Or Equal?(x=w2109, y=w2102) -> (x >= y?=w2111:bool)
                    n1100 = case shown="True" w2111 {
                      tunnel: w2106 -> [w2121 _]
                      tunnel: w2105 -> [w2120 _]
                      tunnel: w2104 -> [w2119 _]
                      tunnel: w2103 -> [w2118 _]
                      frame True {
                        n1101 = stacked-sequence {
                          tunnel: w2121 -> [w2125 _]
                          tunnel: w2120 -> [w2123 w2129]
                          tunnel: w2119 -> [_ w2132]
                          tunnel: w2118 -> [w2122 _]
                          frame #0 {
                            n1102 = Build Array(w2123) -> (w2126:string[])
                            n1103 = Build Array(w2125) -> (w2124:dbl[])
                            n1104 = TDMS Write(0:w2122, 5:"TEST PASS", 7:w2126, 9:w2124) -> (15:w2128:errorcluster)  [unwired: 2 in, 3 out]
                            n1105 = local write "data file error"(w2128) -> ()
                          }
                          frame #1 {
